vi "rszvl_core_global.vi"() -> ()   [LabVIEW 2014] (continued)
CH18,CH19,CH20\r\nSegment: SEG1,SEG2,SEG3,SEG4,SEG5,SEG6,SEG7,SEG8,SEG9,SEG10,SEG11,SEG12,SEG13,SEG14,SEG15,SEG16,SEG17,SEG18,SEG19,SEG20\r\n\nRemote-control command(s):\n[SENSe<Ch>:]SEGMent<Seg>:FREQuency:CENTer?", "Flags"={"OPC Wait"=FALSE, "Dont check status"=FALSE, "*WAI"=FALSE}, "Check Status Callback"=""}, {"Level"=3, "Descriptive Name"="NWA Segment Get Frequency Span", "Class Only"=FALSE, "Data Type"=1, "Access"=0, "Identifier"="RSZVL_ATTR_NWA_SEGMENT_GET_FREQ_SPAN", "Range Table"="", "Command"="SENS{Channel}:SEGM{Segment}:FREQ:SPAN?", "Read Callback"="", "Write Callback"="", "Range Callback"="", "Check Callback"="", "Rngtable Callback"="", "Coerce Callback"="", "User Callback"="", "Supported Models"="", "Instrument Options"="", "Repeated Capabilities"="", "Restricted Repeated Capabilities"="", "Help"="This attribute returns the width of the frequency range of sweep segment no. <Seg>.\n\nAvailable Repeated Capabilities:\nChannel: CH1,CH2,CH3,CH4,CH5,CH6,CH7,CH8,CH9,CH10,CH11,CH12,CH13,CH14,CH15,CH16,CH17,CH18,CH19,CH20\r\nSegment: SEG1,SEG2,SEG3,SEG4,SEG5,SEG6,SEG7,SEG8,SEG9,SEG10,SEG11,SEG12,SEG13,SEG14,SEG15,SEG16,SEG17,SEG18,SEG19,SEG20\r\n\nRemote-control command(s):\n[SENSe<Ch>:]SEGMent<Seg>:FREQuency:SPAN?", "Flags"={"OPC Wait"=FALSE, "Dont check status"=FALSE, "*WAI"=FALSE}, "Check Status Callback"=""}, {"Level"=3, "Descriptive Name"="NWA Store Segment", "Class Only"=FALSE, "Data Type"=2, "Access"=1, "Identifier"="RSZVL_ATTR_NWA_STORE_SEGMENT", "Range Table"="", "Command"="MMEM:STOR:SEGM {Channel},", "Read Callback"="", "Write Callback"="rszvl_quotedString_WriteCallback.vi", "Range Callback"="", "Check Callback"="", "Rngtable Callback"="", "Coerce Callback"="", "User Callback"="", "Supported Models"="", "Instrument Options"="", "Repeated Capabilities"="", "Restricted Repeated Capabilities"="", "Help"="This attribute saves the sweep segment definition of a specified channel to a sweep segment file.\n\nAvailable Repeated Capabilities:\nChannel: CH1,CH2,CH3,CH4,CH5,CH6,CH7,CH8,CH9,CH10,CH11,CH12,CH13,CH14,CH15,CH16,CH17,CH18,CH19,CH20\r\n\nRemote-control command(s):\nMMEMory:STORe:SEGMent <Ch>, '<file_name>'", "Flags"={"OPC Wait"=FALSE, "Dont check status"=FALSE, "*WAI"=FALSE}, "Check Status Callback"=""}, {"Level"=3, "Descriptive Name"="NWA Load Segment", "Class Only"=FALSE, "Data Type"=2, "Access"=1, "Identifier"="RSZVL_ATTR_NWA_LOAD_SEGMENT", "Range Table"="", "Command"="MMEM:LOAD:SEGM {Channel},", "Read Callback"="", "Write Callback"="rszvl_quotedString_WriteCallback.vi", "Range Callback"="", "Check Callback"="", "Rngtable Callback"="", "Coerce Callback"="", "User Callback"="", "Supported Models"="", "Instrument Options"="", "Repeated Capabilities"="", "Restricted Repeated Capabilities"="", "Help"="This attribute loads a sweep segment definition from a specified file and assigns it to a specified channel.\n\nAvailable Repeated Capabilities:\nChannel: CH1,CH2,CH3,CH4,CH5,CH6,CH7,CH8,CH9,CH10,CH11,CH12,CH13,CH14,CH15,CH16,CH17,CH18,CH19,CH20\r\n\nRemote-control command(s):\nMMEMory:LOAD:SEGMent <Ch>,'<file_name>'", "Flags"={"OPC Wait"=FALSE, "Dont check status"=FALSE, "*WAI"=FALSE}, "Check Status Callback"=""}, {"Level"=1, "Descriptive Name"="NWA Correction", "Class Only"=TRUE, "Data Type"=0, "Access"=0, "Identifier"="", "Range Table"="", "Command"="", "Read Callback"="", "Write Callback"="", "Range Callback"="", "Check Callback"="", "Rngtable Callback"="", "Coerce Callback"="", "User Callback"="", "Supported Models"="", "Instrument Options"="", "Repeated Capabilities"="", "Restricted Repeated Capabilities"="", "Help"="(1) NWA Delete Correction:\nThis attribute deletes a system error correction data set stored in the cal pool (cal group file).\n\n(2) NWA Store Correction:\nThis attribute copies the correction data of channel <Ch> to the cal pool, generating a new correction data file (cal group). The file has the extension *.calkit and is stored in the C:\\Rohde&Schwarz\\NWA\\Calibration\\Data directory.\n\n(3) NWA Load Correction:\nThis attribute applies a system error correction data set stored in the cal pool (cal group file) to channel no. <Ch>.\n\n(4) NWA Resolve Correction:\nThis attribute resolves the link between channel <Ch> and the correction data set (cal group file) so that the channel uses its previous correction data. \n\n(5) NWA Calibration Keep Meas Data:\nThis attribute activates or deactivates the calibration mode where the raw measurement data of the standards is stored after the calibration is completed. The setting is valid for the current calibration, where it overwrites the global setting ([SENSe<Ch>:]CORRection:COLLect[:ACQuire]:RSAVe:DEFault). A new calibration deletes the calibration data acquired in previous calibrations.\n\n(6) NWA Calibration Keep Meas Data Default:\nThis attribute activates or deactivates the calibration mode where the raw measurement data of the standards is stored after the calibration is completed. The setting remains valid for all subsequent calibrations until it is changed explicitly. A new calibration deletes the calibration data acquired in previous calibrations.\n\n(7) NWA Export Cal Data To Touchstone File:\nThis attribute converts the calibration data of the standards in the active calibration unit to Touchstone format and copies it to the specified directory.\n\n(8) NWA Connector Type:\nThis attribute selects a connector type at a specified port <port_no> and its gender.\n\n(9) NWA Same Connectors At Ports:\nThis attribute qualifies whether the connector types at the analyzer ports (but not their gender) are equal or independent.\n\n(10) NWA Delete User Defined Connector Type:\nThis attribute deletes a user-defined connector type named '<conn_name>'.\n\n(11) NWA Get Calibration Data Parameters:\nThis attribute returns the sweep settings of the active system error correction for channel <Ch>.\n\n(12) NWA Get Calibration Date:\nThis attribute returns the date and time when the active system error correction data for channel <Ch> was acquired. \n\n(13) NWA Factory Calibration State:\nThis attribute enables or disables the factory calibration for a particular channel.\n\n(14) NWA Calibration Lists (Class):\nPut a help here\n\n(15) NWA Calibration Kits (Class):\nPut a help here\n\n(16) NWA Offset (Class):\nPut a help here", "Flags"={"OPC Wait"=FALSE, "Dont check status"=FALSE, "*WAI"=FALSE}, "Check Status Callback"=""}, {"Level"=2, "Descriptive Name"="NWA Correction State", "Class Only"=FALSE, "Data Type"=3, "Access"=2, "Identifier"="RSZVL_ATTR_NWA_CORRECTION_STATE", "Range Table"="", "Command"="SENS{Channel}:CORR:STAT", "Read Callback"="", "Write Callback"="", "Range Callback"="", "Check Callback"="", "Rngtable Callback"="", "Coerce Callback"="", "User Callback"="", "Supported Models"="", "Instrument Options"="", "Repeated Capabilities"="", "Restricted Repeated Capabilities"="", "Help"="This attribute enables or disables the system error correction for channel <Ch>.\n\nAvailable Repeated Capabilities:\nChannel: CH1,CH2,CH3,CH4,CH5,CH6,CH7,CH8,CH9,CH10,CH11,CH12,CH13,CH14,CH15,CH16,CH17,CH18,CH19,CH20\r\n\nRemote-control command(s):\n[SENSe<Ch>:]CORRection[:STATe] ON | OFF", "Flags"={"OPC Wait"=FALSE, "Dont check status"=FALSE, "*WAI"=FALSE}, "Check Status Callback"=""}, {"Level"=2, "Descriptive Name"="NWA Delete Correction", "Class Only"=FALSE, "Data Type"=2, "Access"=1, "Identifier"="RSZVL_ATTR_NWA_CORRECTION_DELETE", "Range Table"="", "Command"="MMEM:DEL:CORR", "Read Callback"="", "Write Callback"="rszvl_quotedString_WriteCallback.vi", "Range Callback"="", "Check Callback"="", "Rngtable Callback"="", "Coerce Callback"="", "User Callback"="", "Supported Models"="", "Instrument Options"="", "Repeated Capabilities"="", "Restricted Repeated Capabilities"="", "Help"="This attribute deletes a system error correction data set stored in the cal pool (cal group file).\n\nAvailable Repeated Capabilities:\nNone\n\nRemote-control command(s):\nMMEMory:DELete:CORRection <file_name>'", "Flags"={"OPC Wait"=FALSE, "Dont check status"=FALSE, "*WAI"=FALSE}, "Check Status Callback"=""}, {"Level"=2, "Descriptive Name"="NWA Store Correction", "Class Only"=FALSE, "Data Type"=2, "Access"=1, "Identifier"="RSZVL_ATTR_NWA_CORRECTION_STORE", "Range Table"="", "Command"="MMEM:STOR:CORR {Channel},", "Read Callback"="", "Write Callback"="rszvl_quotedString_WriteCallback.vi", "Range Callback"="", "Check Callback"="", "Rngtable Callback"="", "Coerce Callback"="", "User Callback"="", "Supported Models"="", "Instrument Options"="", "Repeated Capabilities"="", "Restricted Repeated Capabilities"="", "Help"="This attribute copies the correction data of channel <Ch> to the cal pool, generating a new correction data file (cal group). The file has the extension *.calkit and is stored in the C:\\Rohde&Schwarz\\NWA\\Calibration\\Data directory.\n\nAvailable Repeated Capabilities:\nChannel: CH1,CH2,CH3,CH4,CH5,CH6,CH7,CH8,CH9,CH10,CH11,CH12,CH13,CH14,CH15,CH16,CH17,CH18,CH19,CH20\r\n\nRemote-control command(s):\nMMEMory:STORe:CORRection <Ch>,'<file_name>'", "Flags"={"OPC Wait"=FALSE, "Dont check status"=FALSE, "*WAI"=FALSE}, "Check Status Callback"=""}, {"Level"=2, "Descriptive Name"="NWA Load Correction", "Class Only"=FALSE, "Data Type"=2, "Access"=1, "Identifier"="RSZVL_ATTR_NWA_CORRECTION_LOAD", "Range Table"="", "Command"="MMEM:LOAD:CORR {Channel},", "Read Callback"="", "Write Callback"="rszvl_quotedString_WriteCallback.vi", "Range Callback"="", "Check Callback"="", "Rngtable Callback"="", "Coerce Callback"="", "User Callback"="", "Supported Models"="", "Instrument Options"="", "Repeated Capabilities"="", "Restricted Repeated Capabilities"="", "Help"="This attribute applies a system error correction data set stored in the cal pool (cal group file) to channel no. <Ch>.\n\nAvailable Repeated Capabilities:\nChannel: CH1,CH2,CH3,CH4,CH5,CH6,CH7,CH8,CH9,CH10,CH11,CH12,CH13,CH14,CH15,CH16,CH17,CH18,CH19,CH20\r\n\nRemote-control command(s):\nMMEMory:LOAD:CORRection <Ch>,'<file_name>'", "Flags"={"OPC Wait"=FALSE, "Dont check status"=FALSE, "*WAI"=FALSE}, "Check Status Callback"=""}, {"Level"=2, "Descriptive Name"="NWA Resolve Correction", "Class Only"=FALSE, "Data Type"=2, "Access"=1, "Identifier"="RSZVL_ATTR_NWA_CORRECTION_RESOLVE", "Range Table"="", "Command"="MMEM:LOAD:CORR:RES {Channel},", "Read Callback"="", "Write Callback"="rszvl_quotedString_WriteCallback.vi", "Range Callback"="", "Check Callback"="", "Rngtable Callback"="", "Coerce Callback"="", "User Callback"="", "Supported Models"="", "Instrument Options"="", "Repeated Capabilities"="", "Restricted Repeated Capabilities"="", "Help"="This attribute resolves the link between channel <Ch> and the correction data set (cal group file) so that the channel uses its previous correction data.\n\nAvailable Repeated Capabilities:\nChannel: CH1,CH2,CH3,CH4,CH5,CH6,CH7,CH8,CH9,CH10,CH11,CH12,CH13,CH14,CH15,CH16,CH17,CH18,CH19,CH20\r\n\nRemote-control command(s):\nMMEMory:LOAD:CORRection:RESolve <Ch>[,'<file_name>']", "Flags"={"OPC Wait"=FALSE, "Dont check status"=FALSE, "*WAI"=FALSE}, "Check Status Callback"=""}, {"Level"=2, "Descriptive Name"="NWA Calibration Keep Meas Data", "Class Only"=FALSE, "Data Type"=3, "Access"=2, "Identifier"="RSZVL_ATTR_NWA_CORR_RSAV", "Range Table"="", "Command"="SENS{Channel}:CORR:COLL:ACQ:RSAV", "Read Callback"="", "Write Callback"="", "Range Callback"="", "Check Callback"="", "Rngtable Callback"="", "Coerce Callback"="", "User Callback"="", "Supported Models"="", "Instrument Options"="", "Repeated Capabilities"="", "Restricted Repeated Capabilities"="", "Help"="This attribute activates or deactivates the calibration mode where the raw measurement data of the standards is stored after the calibration is completed. The setting is valid for the current calibration, where it overwrites the global setting ([SENSe<Ch>:]CORRection:COLLect[:ACQuire]:RSAVe:DEFault). A new calibration deletes the calibration data acquired in previous calibrations.\n\nAvailable Repeated Capabilities:\nChannel: CH1,CH2,CH3,CH4,CH5,CH6,CH7,CH8,CH9,CH10,CH11,CH12,CH13,CH14,CH15,CH16,CH17,CH18,CH19,CH20\r\n\nRemote-control command(s):\n[SENSe<Ch>:]CORRection:COLLect[:ACQuire]:RSAVe ON | OFF", "Flags"={"OPC Wait"=FALSE, "Dont check status"=FALSE, "*WAI"=FALSE}, "Check Status Callback"=""}, {"Level"=2, "Descriptive Name"="NWA Calibration Keep Meas Data Default", "Class Only"=FALSE, "Data Type"=3, "Access"=2, "Identifier"="RSZVL_ATTR_NWA_CORR_RSAV_DEFAULT", "Range Table"="", "Command"="SENS{Channel}:CORR:COLL:ACQ:RSAV:DEF", "Read Callback"="", "Write Callback"="", "Range Callback"="", "Check Callback"="", "Rngtable Callback"="", "Coerce Callback"="", "User Callback"="", "Supported Models"="", "Instrument Options"="", "Repeated Capabilities"="", "Restricted Repeated Capabilities"="", "Help"="This attribute activates or deactivates the calibration mode where the raw measurement data of the standards is stored after the calibration is completed. The setting remains valid for all subsequent calibrations until it is changed explicitly. A new calibration deletes the calibration data acquired in previous calibrations.\n\nAvailable Repeated Capabilities:\nChannel: CH1,CH2,CH3,CH4,CH5,CH6,CH7,CH8,CH9,CH10,CH11,CH12,CH13,CH14,CH15,CH16,CH17,CH18,CH19,CH20\r\n\nRemote-control command(s):\n[SENSe<Ch>:]CORRection:COLLect[:ACQuire]:RSAVe:DEFault ON | OFF", "Flags"={"OPC Wait"=FALSE, "Dont check status"=FALSE, "*WAI"=FALSE}, "Check Status Callback"=""}, {"Level"=2, "Descriptive Name"="NWA Export Cal Data To Touchstone File", "Class Only"=FALSE, "Data Type"=2, "Access"=1, "Identifier"="RSZVL_ATTR_NWA_CORR_EXP_DATA_TOUCH_FILE", "Range Table"="", "Command"="MMEM:AKAL:FACT:CONV", "Read Callback"="", "Write Callback"="rszvl_quotedString_WriteCallback.vi", "Range Callback"="", "Check Callback"="", "Rngtable Callback"="", "Coerce Callback"="", "User Callback"="", "Supported Models"="", "Instrument Options"="", "Repeated Capabilities"="", "Restricted Repeated Capabilities"="", "Help"="This attribute converts the calibration data of the standards in the active calibration unit to Touchstone format and copies it to the specified directory.\n\nAvailable Repeated Capabilities:\nNone\n\nRemote-control command(s):\nMMEMory:AKAL:FACTory:CONVersion '<directory_name>'", "Flags"={"OPC Wait"=FALSE, "Dont check status"=FALSE, "*WAI"=FALSE}, "Check Status Callback"=""}, {"Level"=2, "Descriptive Name"="NWA Connector Type", "Class Only"=FALSE, "Data Type"=0, "Access"=2, "Identifier"="RSZVL_ATTR_NWA_CORR_CONN_TYPE", "Range Table"="rszvl_rngNWAConnectorType", "Command"="SENS{Channel}:CORR:COLL:CONN{Port}", "Read Callback"="", "Write Callback"="", "Range Callback"="", "Check Callback"="", "Rngtable Callback"="", "Coerce Callback"="", "User Callback"="", "Supported Models"="", "Instrument Options"="", "Repeated Capabilities"="", "Restricted Repeated Capabilities"="", "Help"="This attribute selects a connector type at a specified port <port_no> and its gender.\n\nAvailable Repeated Capabilities:\nChannel: CH1,CH2,CH3,CH4,CH5,CH6,CH7,CH8,CH9,CH10,CH11,CH12,CH13,CH14,CH15,CH16,CH17,CH18,CH19,CH20\r\nPort: P1,P2,P3,P4,P5,P6,P7,P8,P9,P10\r\n\nRemote-control command(s):\n[SENSe<Ch>:]CORRection:COLLect:CONNection<port_no> N50FEMALE | N50MALE | N75FEMALE | N75MALE | PC7 | PC35FEMALE | PC35MALE | PC292FEMALE | PC292MALE | UFEMALE1 | UMALE1 | UFEMALE2 | UMALE2", "Flags"={"OPC Wait"=FALSE, "Dont check status"=FALSE, "*WAI"=FALSE}, "Check Status Callback"=""}, {"Level"=2, "Descriptive Name"="NWA Same Connectors At Ports", "Class Only"=FALSE, "Data Type"=0, "Access"=2, "Identifier"="RSZVL_ATTR_NWA_CORR_CONN_PORTS", "Range Table"="rszvl_rngNWASameConnectorsAtPorts", "Command"="SENS{Channel}:CORR:COLL:CONN:PORT", "Read Callback"="", "Write Callback"="", "Range Callback"="", "Check Callback"="", "Rngtable Callback"="", "Coerce Callback"="", "User Callback"="", "Supported Models"="", "Instrument Options"="", "Repeated Capabilities"="", "Restricted Repeated Capabilities"="", "Help"="This attribute qualifies whether the connector types at the analyzer ports (but not their gender) are equal or independent.\n\nAvailable Repeated Capabilities:\nChannel: CH1,CH2,CH3,CH4,CH5,CH6,CH7,CH8,CH9,CH10,CH11,CH12,CH13,CH14,CH15,CH16,CH17,CH18,CH19,CH20\r\n\nRemote-control command(s):\n[SENSe<Ch>:]CORRection:COLLect:CONNection:PORTs ALL | SINGle", "Flags"={"OPC Wait"=FALSE, "Dont check status"=FALSE, "*WAI"=FALSE}, "Check Status Callback"=""}, {"Level"=2, "Descriptive Name"="NWA Delete User Defined Connector Type", "Class Only"=FALSE, "Data Type"=2, "Access"=1, "Identifier"="RSZVL_ATTR_NWA_CORR_DELETE_USER_CONN", "Range Table"="", "Command"="SENS{Channel}:CORR:CONN:DEL", "Read Callback"="", "Write Callback"="rszvl_quotedString_WriteCallback.vi", "Range Callback"="", "Check Callback"="", "Rngtable Callback"="", "Coerce Callback"="", "User Callback"="", "Supported Models"="", "Instrument Options"="", "Repeated Capabilities"="", "Restricted Repeated Capabilities"="", "Help"="This attribute deletes a user-defined connector type named '<conn_name>'.\n\nAvailable Repeated Capabilities:\nChannel: CH1,CH2,CH3,CH4,CH5,CH6,CH7,CH8,CH9,CH10,CH11,CH12,CH13,CH14,CH15,CH16,CH17,CH18,CH19,CH20\r\n\nRemote-control command(s):\n[SENSe<Ch>:]CORRection:CONNection:DELete '<conn_name>'", "Flags"={"OPC Wait"=FALSE, "Dont check status"=FALSE, "*WAI"=FALSE}, "Check Status Callback"=""}, {"Level"=2, "Descriptive Name"="NWA Get Calibration State", "Class Only"=FALSE, "Data Type"=0, "Access"=0, "Identifier"="RSZVL_ATTR_NWA_CORR_GET_CAL_STATE", "Range Table"="rszvl_rngNWAGetCalState", "Command"="SENS{Channel}:CORR:SST?", "Read Callback"="rszvl_quotedInt_ReadCallback.vi", "Write Callback"="", "Range Callback"="", "Check Callback"="", "Rngtable Callback"="", "Coerce Callback"="", "User Callback"="", "Supported Models"="", "Instrument Options"="", "Repeated Capabilities"="", "Restricted Repeated Capabilities"="", "Help"="This attribute returns the state of the active system error correction for channel <Ch>.\n\nAvailable Repeated Capabilities:\nChannel: CH1,CH2,CH3,CH4,CH5,CH6,CH7,CH8,CH9,CH10,CH11,CH12,CH13,CH14,CH15,CH16,CH17,CH18,CH19,CH20\r\n\nRemote-control command(s):\n[SENSe<Ch>:]CORRection:SSTate?", "Flags"={"OPC Wait"=FALSE, "Dont check status"=FALSE, "*WAI"=FALSE}, "Check Status Callback"=""}, {"Level"=2, "Descriptive Name"="NWA Get Calibration Data Parameters", "Class Only"=FALSE, "Data Type"=2, "Access"=0, "Identifier"="RSZVL_ATTR_NWA_CORR_GET_CAL_DATA_PARAMS", "Range Table"="", "Command"="SENS{Channel}:CORR:DATA:PAR?", "Read Callback"="", "Write Callback"="", "Range Callback"="", "Check Callback"="", "Rngtable Callback"="", "Coerce Callback"="", "User Callback"="", "Supported Models"="", "Instrument Options"="", "Repeated Capabilities"="", "Restricted Repeated Capabilities"="", "Help"="This attribute returns the sweep settings of the active system error correction for channel <Ch>.\n\nAvailable Repeated Capabilities:\nChannel: CH1,CH2,CH3,CH4,CH5,CH6,CH7,CH8,CH9,CH10,CH11,CH12,CH13,CH14,CH15,CH16,CH17,CH18,CH19,CH20\r\n\nRemote-control command(s):\n[SENSe<Ch>:]CORRection:DATA:PARameter?", "Flags"={"OPC Wait"=FALSE, "Dont check status"=FALSE, "*WAI"=FALSE}, "Check Status Callback"=""}, {"Level"=2, "Descriptive Name"="NWA Get Calibration Date", "Class Only"=FALSE, "Data Type"=2, "Access"=0, "Identifier"="RSZVL_ATTR_NWA_CORR_GET_CAL_DATE", "Range Table"="", "Command"="SENS{Channel}:CORR:DATE?", "Read Callback"="rszvl_quotedString_ReadCallback.vi", "Write Callback"="", "Range Callback"="", "Check Callback"="", "Rngtable Callback"="", "Coerce Callback"="", "User Callback"="", "Supported Models"="", "Instrument Options"="", "Repeated Capabilities"="", "Restricted Repeated Capabilities"="", "Help"="This attribute returns the date and time when the active system error correction data for channel <Ch> was acquired.\n\nAvailable Repeated Capabilities:\nChannel: CH1,CH2,CH3,CH4,CH5,CH6,CH7,CH8,CH9,CH10,CH11,CH12,CH13,CH14,CH15,CH16,CH17,CH18,CH19,CH20\r\n\nRemote-control command(s):\n[SENSe<Ch>:]CORRection:DATE?", "Flags"={"OPC Wait"=FALSE, "Dont check status"=FALSE, "*WAI"=FALSE}, "Check Status Callback"=""}, {"Level"=2, "Descriptive Name"="NWA Factory Calibration State", "Class Only"=FALSE, "Data Type"=3, "Access"=2, "Identifier"="RSZVL_ATTR_NWA_CORR_FACT_CAL_STATE", "Range Table"="", "Command"="SENS{Channel}:CORR:FACT:STAT", "Read Callback"="", "Write Callback"="", "Range Callback"="", "Check Callback"="", "Rngtable Callback"="", "Coerce Callback"="", "User Callback"="", "Supported Models"="", "Instrument Options"="", "Repeated Capabilities"="", "Restricted Repeated Capabilities"="", "Help"="This attribute enables or disables the factory calibration for a particular channel.\n\nAvailable Repeated Capabilities:\nChannel: CH1,CH2,CH3,CH4,CH5,CH6,CH7,CH8,CH9,CH10,CH11,CH12,CH13,CH14,CH15,CH16,CH17,CH18,CH19,CH20\r\n\nRemote-control command(s):\n[SENSe<Ch>:]CORRection:FACTory[:STATe] ON | OFF", "Flags"={"OPC Wait"=FALSE, "Dont check status"=FALSE, "*WAI"=FALSE}, "Check Status Callback"=""}, {"Level"=2, "Descriptive Name"="NWA Automatic Calibration", "Class Only"=TRUE, "Data Type"=0, "Access"=0, "Identifier"="", "Range Table"="", "Command"="", "Read Callback"="", "Write Callback"="", "Range Callback"="", "Check Callback"="", "Rngtable Callback"="", "Coerce Callback"="", "User Callback"="", "Supported Models"="", "Instrument Options"="", "Repeated Capabilities"="", "Restricted Repeated Capabilities"="", "Help"="Put a help here", "Flags"={"OPC Wait"=FALSE, "Dont check status"=FALSE, "*WAI"=FALSE}, "Check Status Callback"=""}, {"Level"=3, "Descriptive Name"="NWA Generate Calibration Kit File", "Class Only"=FALSE, "Data Type"=2, "Access"=1, "Identifier"="RSZVL_ATTR_NWA_GENERATE_CALIBRATION_KIT_FILE", "Range Table"="", "Command"="SENS:CORR:COLL:AUTO:CKIT", "Read Callback"="", "Write Callback"="", "Range Callback"="", "Check Callback"="", "Rngtable Callback"="", "Coerce Callback"="", "User Callback"="", "Supported Models"="", "Instrument Options"="", "Repeated Capabilities"="", "Restricted Repeated Capabilities"="", "Help"="This attribute generates a cal kit file with the specified name containing the cal kit data of the active calibration unit. The cal kit file can be stored in the calibration unit or written to a directory on the analyzer.\n\nAvailable Repeated Capabilities:\nNone\n\nRemote-control command(s):\n[SENSe<Ch>:]CORRection:COLLect:AUTO:CKIT", "Flags"={"OPC Wait"=FALSE, "Dont check status"=FALSE, "*WAI"=FALSE}, "Check Status Callback"=""}, {"Level"=3, "Descriptive Name"="NWA Active Calibration Unit", "Class Only"=FALSE, "Data Type"=2, "Access"=2, "Identifier"="RSZVL_ATTR_NWA_ACTIVE_CALIBRATION_UNIT", "Range Table"="", "Command"="SYST:COMM:RDEV:AKAL:ADDR", "Read Callback"="rszvl_quotedString_ReadCallback.vi", "Write Callback"="rszvl_quotedString_WriteCallback.vi", "Range Callback"="", "Check Callback"="", "Rngtable Callback"="", "Coerce Callback"="", "User Callback"="", "Supported Models"="", "Instrument Options"="", "Repeated Capabilities"="", "Restricted Repeated Capabilities"="", "Help"="This attribute selects one of the USB-connected calibration units for calibration. This function is not necessary if only one cal unit is connected.\n\nAvailable Repeated Capabilities:\nNone\n\nRemote-control command(s):\nSYSTem:COMMunicate:RDEVice:AKAL:ADDRess", "Flags"={"OPC Wait"=FALSE, "Dont check status"=FALSE, "*WAI"=FALSE}, "Check Status Callback"=""}, {"Level"=3, "Descriptive Name"="NWA Get All Calibration Units", "Class Only"=FALSE, "Data Type"=2, "Access"=0, "Identifier"="RSZVL_ATTR_NWA_GET_ALL_CALIBRATION_UNITS", "Range Table"="", "Command"="SYST:COMM:RDEV:AKAL:ADDR:ALL?", "Read Callback"="rszvl_quotedString_ReadCallback.vi", "Write Callback"="", "Range Callback"="", "Check Callback"="", "Rngtable Callback"="", "Coerce Callback"="", "User Callback"="", "Supported Models"="", "Instrument Options"="", "Repeated Capabilities"="", "Restricted Repeated Capabilities"="", "Help"="This attribute returns the names (USB addresses) of all connected calibration units.\n\nAvailable Repeated Capabilities:\nNone\n\nRemote-control command(s):\nSYSTem:COMMunicate:RDEVice:AKAL:ADDRess:ALL?", "Flags"={"OPC Wait"=FALSE, "Dont check status"=FALSE, "*WAI"=FALSE}, "Check Status Callback"=""}, {"Level"=3, "Descriptive Name"="NWA Export Calibration Data To Touchstone Format", "Class Only"=FALSE, "Data Type"=2, "Access"=1, "Identifier"="RSZVL_ATTR_NWA_EXPORT_CALIBRATION_DATA_TO_TOUCHSTONE_FORMAT", "Range Table"="", "Command"="MMEM:AKAL:FACT:CONV", "Read Callback"="", "Write Callback"="", "Range Callback"="", "Check Callback"="", "Rngtable Callback"="", "Coerce Callback"="", "User Callback"="", "Supported Models"="", "Instrument Options"="", "Repeated Capabilities"="", "Restricted Repeated Capabilities"="", "Help"="This attribute converts the calibration data of the standards in the active calibration unit to Touchstone format and copies it to the specified directory.\n\nAvailable Repeated Capabilities:\nNone\n\nRemote-control command(s):\nMMEMory:AKAL:FACTory:CONVersion", "Flags"={"OPC Wait"=FALSE, "Dont check status"=FALSE, "*WAI"=FALSE}, "Check Status Callback"=""}, {"Level"=2, "Descriptive Name"="NWA Calibration Lists", "Class Only"=TRUE, "Data Type"=0, "Access"=0, "Identifier"="", "Range Table"="", "Command"="", "Read Callback"="", "Write Callback"="", "Range Callback"="", "Check Callback"="", "Rngtable Callback"="", "Coerce Callback"="", "User Callback"="", "Supported Models"="", "Instrument Options"="", "Repeated Capabilities"="", "Restricted Repeated Capabilities"="", "Help"="Put a help here", "Flags"={"OPC Wait"=FALSE, "Dont check status"=FALSE, "*WAI"=FALSE}, "Check Status Callback"=""}, {"Level"=3, "Descriptive Name"="NWA Save Calibration Data", "Class Only"=FALSE, "Data Type"=4, "Access"=1, "Identifier"="RSZVL_ATTR_NWA_CORR_SAVE_CAL_DATA", "Range Table"="", "Command"="SENS{Channel}:CORR:COLL:SAVE:SEL", "Read Callback"="", "Write Callback"="", "Range Callback"="", "Check Callback"="", "Rngtable Callback"="", "Coerce Callback"="", "User Callback"="", "Supported Models"="", "Instrument Options"="", "Repeated Capabilities"="", "Restricted Repeated Capabilities"="", "Help"="This attribute calculates the system error correction data from the acquired measurement results ([SENSe<Ch>:]CORRection:COLLect[:ACQuire]:SELected), stores them and applies them to the calibrated channel <Ch>. To avoid incompatibilities, older system error correction data is deleted unless it has been transferred into a cal pool (MMEMory:STORe:CORRection <Ch>, '<file_name>').\n\nAvailable Repeated Capabilities:\nChannel: CH1,CH2,CH3,CH4,CH5,CH6,CH7,CH8,CH9,CH10,CH11,CH12,CH13,CH14,CH15,CH16,CH17,CH18,CH19,CH20\r\n\nRemote-control command(s):\n[SENSe<Ch>:]CORRection:COLLect:SAVE:SELected", "Flags"={"OPC Wait"=FALSE, "Dont check status"=FALSE, "*WAI"=FALSE}, "Check Status Callback"=""}, {"Level"=3, "Descriptive Name"="NWA Generate Default Cal Data", "Class Only"=FALSE, "Data Type"=4, "Access"=1, "Identifier"="RSZVL_ATTR_NWA_CORR_SAVE_DEFAULT_DATA", "Range Table"="", "Command"="SENS{Channel}:CORR:COLL:SAVE:SEL:DEF", "Read Callback"="", "Write Callback"="", "Range Callback"="", "Check Callback"="", "Rngtable Callback"="", "Coerce Callback"="", "User Callback"="", "Supported Models"="", "Instrument Options"="", "Repeated Capabilities"="", "Restricted Repeated Capabilities"="", "Help"="This attribute generates a set of default system error correction data for the selected ports and calibration type. The default data set corresponds to a test setup which does not introduce any systematic errors.\n\nAvailable Repeated Capabilities:\nChannel: CH1,CH2,CH3,CH4,CH5,CH6,CH7,CH8,CH9,CH10,CH11,CH12,CH13,CH14,CH15,CH16,CH17,CH18,CH19,CH20\r\n\nRemote-control command(s):\n[SENSe<Ch>:]CORRection:COLLect:SAVE:SELected:DEFault", "Flags"={"OPC Wait"=FALSE, "Dont check status"=FALSE, "*WAI"=FALSE}, "Check Status Callback"=""}, {"Level"=3, "Descriptive Name"="NWA Delete Calibration Data", "Class Only"=FALSE, "Data Type"=2, "Access"=1, "Identifier"="RSZVL_ATTR_NWA_CORR_DELETE_CAL_DATA", "Range Table"="", "Command"="SENS{Channel}:CORR:COLL:DEL", "Read Callback"="", "Write Callback"="rszvl_quotedString_WriteCallback.vi", "Range Callback"="", "Check Callback"="", "Rngtable Callback"="", "Coerce Callback"="", "User Callback"="", "Supported Models"="", "Instrument Options"="", "Repeated Capabilities"="", "Restricted Repeated Capabilities"="", "Help"="This attribute deletes system error correction data generated and stored previously.\n\nAvailable Repeated Capabilities:\nChannel: CH1,CH2,CH3,CH4,CH5,CH6,CH7,CH8,CH9,CH10,CH11,CH12,CH13,CH14,CH15,CH16,CH17,CH18,CH19,CH20\r\n\nRemote-control command(s):\n[SENSe<Ch>:]CORRection:COLLect:DELete '<cal_name>'", "Flags"={"OPC Wait"=FALSE, "Dont check status"=FALSE, "*WAI"=FALSE}, "Check Status Callback"=""}, {"Level"=3, "Descriptive Name"="NWA Delete Last Calibration Data", "Class Only"=FALSE, "Data Type"=4, "Access"=1, "Identifier"="RSZVL_ATTR_NWA_CORR_DELETE_CAL_DATA_LAST", "Range Table"="", "Command"="SENS{Channel}:CORR:COLL:DEL", "Read Callback"="", "Write Callback"="", "Range Callback"="", "Check Callback"="", "Rngtable Callback"="", "Coerce Callback"="", "User Callback"="", "Supported Models"="", "Instrument Options"="", "Repeated Capabilities"="", "Restricted Repeated Capabilities"="", "Help"="This attribute deletes system error correction data generated and stored previously.\n\nAvailable Repeated Capabilities:\nChannel: CH1,CH2,CH3,CH4,CH5,CH6,CH7,CH8,CH9,CH10,CH11,CH12,CH13,CH14,CH15,CH16,CH17,CH18,CH19,CH20\r\n\nRemote-control command(s):\n[SENSe<Ch>:]CORRection:COLLect:DELete", "Flags"={"OPC Wait"=FALSE, "Dont check status"=FALSE, "*WAI"=FALSE}, "Check Status Callback"=""}, {"Level"=2, "Descriptive Name"="NWA Calibration Kits", "Class Only"=TRUE, "Data Type"=0, "Access"=0, "Identifier"="", "Range Table"="", "Command"="", "Read Callback"="", "Write Callback"="", "Range Callback"="", "Check Callback"="", "Rngtable Callback"="", "Coerce Callback"="", "User Callback"="", "Supported Models"="", "Instrument Options"="", "Repeated Capabilities"="", "Restricted Repeated Capabilities"="", "Help"="Put a help here", "Flags"={"OPC Wait"=FALSE, "Dont check status"=FALSE, "*WAI"=FALSE}, "Check Status Callback"=""}, {"Level"=3, "Descriptive Name"="NWA Load Calibration Kit", "Class Only"=FALSE, "Data Type"=2, "Access"=1, "Identifier"="RSZVL_ATTR_NWA_LOAD_CAL_KIT", "Range Table"="", "Command"="MMEM:LOAD:CKIT", "Read Callback"="", "Write Callback"="rszvl_quotedString_WriteCallback.vi", "Range Callback"="", "Check Callback"="", "Rngtable Callback"="", "Coerce Callback"="", "User Callback"="", "Supported Models"="", "Instrument Options"="", "Repeated Capabilities"="", "Restricted Repeated Capabilities"="", "Help"="This attribute loads cal kit data from a specified NWA cal kit file.\n\nAvailable Repeated Capabilities:\nNone\n\nRemote-control command(s):\nMMEMory:LOAD:CKIT '<file_name>'", "Flags"={"OPC Wait"=FALSE, "Dont check status"=FALSE, "*WAI"=FALSE}, "Check Status Callback"=""}, {"Level"=2, "Descriptive Name"="NWA Offset", "Class Only"=TRUE, "Data Type"=0, "Access"=0, "Identifier"="", "Range Table"="", "Command"="", "Read Callback"="", "Write Callback"="", "Range Callback"="", "Check Callback"="", "Rngtable Callback"="", "Coerce Callback"="", "User Callback"="", "Supported Models"="", "Instrument Options"="", "Repeated Capabilities"="", "Restricted Repeated Capabilities"="", "Help"="Put a help here", "Flags"={"OPC Wait"=FALSE, "Dont check status"=FALSE, "*WAI"=FALSE}, "Check Status Callback"=""}, {"Level"=3, "Descriptive Name"="NWA Offset Electrical Length", "Class Only"=FALSE, "Data Type"=1, "Access"=2, "Identifier"="RSZVL_ATTR_NWA_OFFSET_ELENGTH", "Range Table"="", "Command"="SENS{Channel}:CORR:EDEL{Port}:ELEN", "Read Callback"="", "Write Callback"="", "Range Callback"="", "Check Callback"="", "Rngtable Callback"="", "Coerce Callback"="", "User Callback"="", "Supported Models"="", "Instrument Options"="", "Repeated Capabilities"="", "Restricted Repeated Capabilities"="", "Help"="This attribute defines the offset parameter for test port <port_no> as an electrical length.\n\nAvailable Repeated Capabilities:\nChannel: CH1,CH2,CH3,CH4,CH5,CH6,CH7,CH8,CH9,CH10,CH11,CH12,CH13,CH14,CH15,CH16,CH17,CH18,CH19,CH20\r\nPort: P1,P2,P3,P4,P5,P6,P7,P8,P9,P10\r\n\nRemote-control command(s):\n[SENSe<Ch>:]CORRection:EDELay<port_no>:ELENgth", "Flags"={"OPC Wait"=FALSE, "Dont check status"=FALSE, "*WAI"=FALSE}, "Check Status Callback"=""}, {"Level"=3, "Descriptive Name"="NWA Offset Permittivity", "Class Only"=FALSE, "Data Type"=1, "Access"=2, "Identifier"="RSZVL_ATTR_NWA_OFFSET_PERMITTIVITY", "Range Table"="", "Command"="SENS{Channel}:CORR:EDEL{Port}:DIEL", "Read Callback"="", "Write Callback"="", "Range Callback"="", "Check Callback"="", "Rngtable Callback"="", "Coerce Callback"="", "User Callback"="", "Supported Models"="", "Instrument Options"="", "Repeated Capabilities"="", "Restricted Repeated Capabilities"="", "Help"="This attribute defines the permittivity for the offset correction at test port <port_no>.\n\nAvailable Repeated Capabilities:\nChannel: CH1,CH2,CH3,CH4,CH5,CH6,CH7,CH8,CH9,CH10,CH11,CH12,CH13,CH14,CH15,CH16,CH17,CH18,CH19,CH20\r\nPort: P1,P2,P3,P4,P5,P6,P7,P8,P9,P10\r\n\nRemote-control command(s):\n[SENSe<Ch>:]CORRection:EDELay<port_no>:DIELectric", "Flags"={"OPC Wait"=FALSE, "Dont check status"=FALSE, "*WAI"=FALSE}, "Check Status Callback"=""}, {"Level"=3, "Descriptive Name"="NWA Offset Mechanical Length", "Class Only"=FALSE, "Data Type"=1, "Access"=2, "Identifier"="RSZVL_ATTR_NWA_OFFSET_DISTANCE", "Range Table"="", "Command"="SENS{Channel}:CORR:EDEL{Port}:DIST", "Read Callback"="", "Write Callback"="", "Range Callback"="", "Check Callback"="", "Rngtable Callback"="", "Coerce Callback"="", "User Callback"="", "Supported Models"="", "Instrument Options"="", "Repeated Capabilities"="", "Restricted Repeated Capabilities"="", "Help"="This attribute defines the offset parameter for test port <port_no> as a mechanical length.\n\nAvailable Repeated Capabilities:\nChannel: CH1,CH2,CH3,CH4,CH5,CH6,CH7,CH8,CH9,CH10,CH11,CH12,CH13,CH14,CH15,CH16,CH17,CH18,CH19,CH20\r\nPort: P1,P2,P3,P4,P5,P6,P7,P8,P9,P10\r\n\nRemote-control command(s):\n[SENSe<Ch>:]CORRection:EDELay<port_no>:DISTance", "Flags"={"OPC Wait"=FALSE, "Dont check status"=FALSE, "*WAI"=FALSE}, "Check Status Callback"=""}, {"Level"=3, "Descriptive Name"="NWA Offset Delay", "Class Only"=FALSE, "Data Type"=1, "Access"=2, "Identifier"="RSZVL_ATTR_NWA_OFFSET_DELAY", "Range Table"="", "Command"="SENS{Channel}:CORR:EDEL{Port}:TIME", "Read Callback"="", "Write Callback"="", "Range Callback"="", "Check Callback"="", "Rngtable Callback"="", "Coerce Callback"="", "User Callback"="", "Supported Models"="", "Instrument Options"="", "Repeated Capabilities"="", "Restricted Repeated Capabilities"="", "Help"="This attribute defines the offset parameter for test port <port_no> as a delay time.\n\nAvailable Repeated Capabilities:\nChannel: CH1,CH2,CH3,CH4,CH5,CH6,CH7,CH8,CH9,CH10,CH11,CH12,CH13,CH14,CH15,CH16,CH17,CH18,CH19,CH20\r\nPort: P1,P2,P3,P4,P5,P6,P7,P8,P9,P10\r\n\nRemote-control command(s):\n[SENSe<Ch>:]CORRection:EDELay<port_no>[:TIME]", "Flags"={"OPC Wait"=FALSE, "Dont check status"=FALSE, "*WAI"=FALSE}, "Check Status Callback"=""}, {"Level"=3, "Descriptive Name"="NWA Offset Auto Length", "Class Only"=FALSE, "Data Type"=4, "Access"=1, "Identifier"="RSZVL_ATTR_NWA_OFFSET_AUTO_LENGTH", "Range Table"="", "Command"="SENS{Channel}:CORR:EDEL{Port}:AUTO ONCE", "Read Callback"="", "Write Callback"="", "Range Callback"="", "Check Callback"="", "Rngtable Callback"="", "Coerce Callback"="", "User Callback"="", "Supported Models"="", "Instrument Options"="", "Repeated Capabilities"="", "Restricted Repeated Capabilities"="", "Help"="The attribute defines the offset parameter for the active test port such that the residual delay of the active trace (defined as the negative derivative of the phase response) is minimized across the entire sweep range.\n\nAvailable Repeated Capabilities:\nChannel: CH1,CH2,CH3,CH4,CH5,CH6,CH7,CH8,CH9,CH10,CH11,CH12,CH13,CH14,CH15,CH16,CH17,CH18,CH19,CH20\r\nPort: P1,P2,P3,P4,P5,P6,P7,P8,P9,P10\r\n\nRemote-control command(s):\n[SENSe<Ch>:]CORRection:EDELay<port_no>:AUTO ONCE", "Flags"={"OPC Wait"=FALSE, "Dont check status"=FALSE, "*WAI"=FALSE}, "Check Status Callback"=""}, {"Level"=3, "Descriptive Name"="NWA Offset Loss", "Class Only"=FALSE, "Data Type"=1, "Access"=2, "Identifier"="RSZVL_ATTR_NWA_OFFSET_LOSS", "Range Table"="rszvl_rngNWAOffsetLoss", "Command"="SENS{Channel}:CORR:LOSS{Port}", "Read Callback"="", "Write Callback"="", "Range Callback"="", "Check Callback"="", "Rngtable Callback"="", "Coerce Callback"="", "User Callback"="", "Supported Models"="", "Instrument Options"="", "Repeated Capabilities"="", "Restricted Repeated Capabilities"="", "Help"="This attribute defines the frequency-independent part (DC value) of the offset loss.\n\nAvailable Repeated Capabilities:\nChannel: CH1,CH2,CH3,CH4,CH5,CH6,CH7,CH8,CH9,CH10,CH11,CH12,CH13,CH14,CH15,CH16,CH17,CH18,CH19,CH20\r\nPort: P1,P2,P3,P4,P5,P6,P7,P8,P9,P10\r\n\nRemote-control command(s):\n[SENSe<Ch>:]CORRection:LOSS<port_no>", "Flags"={"OPC Wait"=FALSE, "Dont check status"=FALSE, "*WAI"=FALSE}, "Check Status Callback"=""}, {"Level"=3, "Descriptive Name"="NWA Offset Loss Offset", "Class Only"=FALSE, "Data Type"=1, "Access"=2, "Identifier"="RSZVL_ATTR_NWA_OFFSET_LOSS_OFFSET", "Range Table"="rszvl_rngNWAOffsetLoss", "Command"="SENS{Channel}:CORR:LOSS{Port}:OFFS", "Read Callback"="", "Write Callback"="", "Range Callback"="", "Check Callback"="", "Rngtable Callback"="", "Coerce Callback"="", "User Callback"="", "Supported Models"="", "Instrument Options"="", "Repeated Capabilities"="", "Restricted Repeated Capabilities"="", "Help"="This attribute defines the offset loss at the reference frequency.\n\nAvailable Repeated Capabilities:\nChannel: CH1,CH2,CH3,CH4,CH5,CH6,CH7,CH8,CH9,CH10,CH11,CH12,CH13,CH14,CH15,CH16,CH17,CH18,CH19,CH20\r\nPort: P1,P2,P3,P4,P5,P6,P7,P8,P9,P10\r\n\nRemote-control command(s):\n[SENSe<Ch>:]CORRection:LOSS<port_no>:OFFSet", "Flags"={"OPC Wait"=FALSE, "Dont check status"=FALSE, "*WAI"=FALSE}, "Check Status Callback"=""}, {"Level"=3, "Descriptive Name"="NWA Offset Loss Frequency", "Class Only"=FALSE, "Data Type"=1, "Access"=2, "Identifier"="RSZVL_ATTR_NWA_OFFSET_LOSS_FREQUENCY", "Range Table"="", "Command"="SENS{Channel}:CORR:LOSS{Port}:FREQ", "Read Callback"="", "Write Callback"="", "Range Callback"="", "Check Callback"="", "Rngtable Callback"="", "Coerce Callback"="", "User Callback"="", "Supported Models"="", "Instrument Options"="", "Repeated Capabilities"="", "Restricted Repeated Capabilities"="", "Help"="This attribute defines the reference frequency for the frequency-dependent part of the offset loss.\n\nAvailable Repeated Capabilities:\nChannel: CH1,CH2,CH3,CH4,CH5,CH6,CH7,CH8,CH9,CH10,CH11,CH12,CH13,CH14,CH15,CH16,CH17,CH18,CH19,CH20\r\nPort: P1,P2,P3,P4,P5,P6,P7,P8,P9,P10\r\n\nRemote-control command(s):\n[SENSe<Ch>:]CORRection:LOSS<port_no>:FREQuency", "Flags"={"OPC Wait"=FALSE, "Dont check status"=FALSE, "*WAI"=FALSE}, "Check Status Callback"=""}, {"Level"=3, "Descriptive Name"="NWA Offset Auto Lenght And Loss", "Class Only"=FALSE, "Data Type"=4, "Access"=1, "Identifier"="RSZVL_ATTR_NWA_OFFSET_AUTO_LENGTH_AND_LOSS", "Range Table"="", "Command"="SENS{Channel}:CORR:LOSS{Port}:AUTO ONCE", "Read Callback"="", "Write Callback"="", "Range Callback"="", "Check Callback"="", "Rngtable Callback"="", "Coerce Callback"="", "User Callback"="", "Supported Models"="", "Instrument Options"="", "Repeated Capabilities"="", "Restricted Repeated Capabilities"="", "Help"="This attribute defines the offset parameters for the active test port such that the residual delay of the active trace (defined as the negative derivative of the phase response) is minimized and the measured 
